vi "Format Gas Params.vi"() -> ()   [LabVIEW 2012]
panel:
  out "错误输出":cluster{"状态":bool, "代码":i32, "源":string}
  in  "错误输入":cluster{"状态":bool, "代码":i32, "源":string}
  out "结果":string="温度： 1.000000\r 气压： 2.000000\r 湿度： 3.000000\r 体积： 4.000000 \r 密度： 5.000000"
  in  "密度":dbl=5.0
  in  "体积":dbl=4.0
  in  "湿度":dbl=3.0
  in  "气压":dbl=2.0
  in  "温度":dbl=1.0
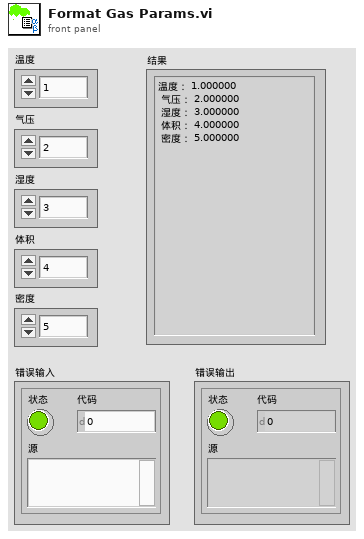
[diagram p1: front panel]
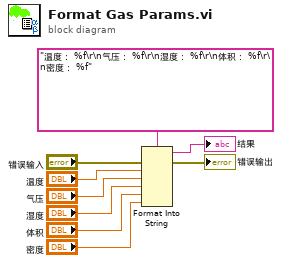
[diagram p0: block diagram]
diagram:
  n1 = Format Into String ("格式化写入字符串")(format string="温度： %f\r\n气压： %f\r\n湿度： %f\r\n体积： %f\r\n密度： %f" ("格式字符串"), error in="错误输入", "温度", "气压", "湿度", "体积", "密度") -> (resulting string=→"结果":string, error out=→"错误输出":errorcluster)  [unwired: 1 in]
